vi "Generate SQL Values.vi"(8 "error in (no error)":errorcluster, 11 "Transaction in":refnum<class "Transaction.lvclass">) -> (0 "error out":errorcluster, 2 "SQL Values":string, 3 "Transaction out":refnum<class "Transaction.lvclass">)   [LabVIEW 2018, in "Transaction.lvclass"]
uses:
  Transaction/Transaction.lvclass
  Transaction/Transaction.lvclass/Transaction.ctl
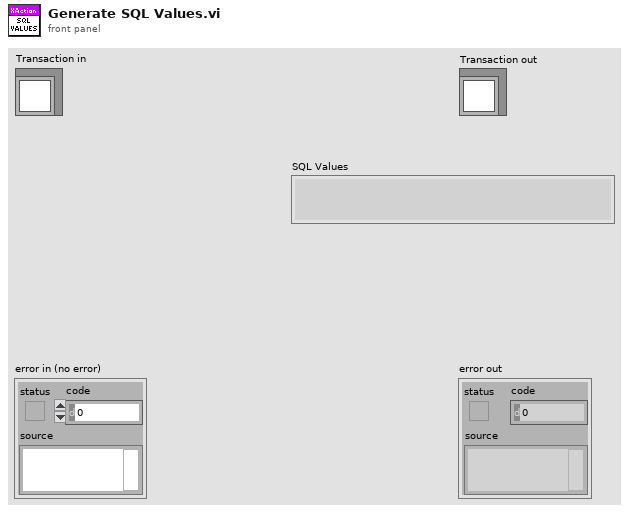
[diagram p1: front panel]
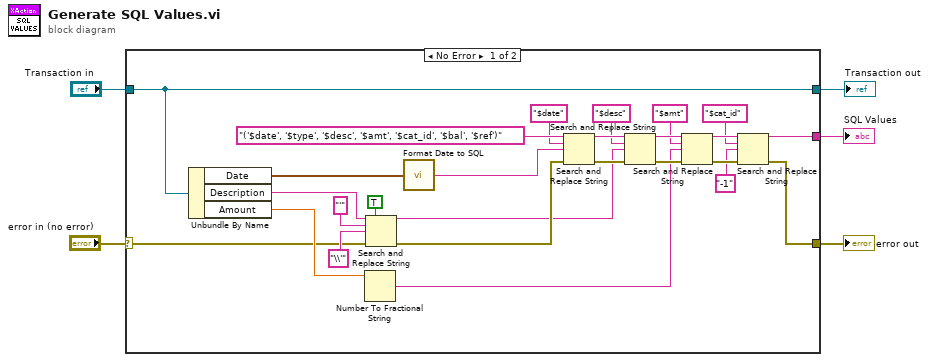
[diagram p0: block diagram]
diagram:
  n1 = case shown="No Error" "error in (no error)" {
    selector: "error in (no error)" -> [w26 w33]
    tunnel: [w13 w33] -> w4
    tunnel: "Transaction in" -> [w25 w32]
    tunnel: [w25 w32] -> w2
    tunnel: [w12 _] -> w1
    frame No Error {
      n2 = Unbundle By Name(w25) -> ("Date"=w24:timestamp, "Description"=w28:string, "Amount"=w27:dbl)
      n3 = Number To Fractional String(number=w27) -> (F-format string=w10:string)  [unwired: 3 in]
      n4 = Search and Replace String(replace all?=TRUE ("replace all? (F)"), input string=w28, search string="'", replace string="\\'", error in=w26) -> (result string=w11:string, error out=w14:errorcluster)  [unwired: 5 out]
      n5 = call "Format Date to SQL.vi"("Date"=w24) -> ("SQL Date"=w21:string)
      n6 = Search and Replace String(input string="('$date', '$type', '$desc', '$amt', '$cat_id', '$bal', '$ref')", search string="$date", replace string=w21, error in=w14) -> (result string=w19:string, error out=w20:errorcluster)  [unwired: 4 in, 2 out]
      n7 = Search and Replace String(input string=w19, search string="$desc", replace string=w11, error in=w20) -> (result string=w18:string, error out=w17:errorcluster)  [unwired: 4 in, 2 out]
      n8 = Search and Replace String(input string=w18, search string="$amt", replace string=w10, error in=w17) -> (result string=w16:string, error out=w15:errorcluster)  [unwired: 4 in, 2 out]
      n9 = Search and Replace String(input string=w16, search string="$cat_id", replace string="-1" ("replace string (\"\")"), error in=w15) -> (result string=w12:string, error out=w13:errorcluster)  [unwired: 4 in, 2 out]
    }
    frame Error {
    }
  }
  "error out" <- w4
  "Transaction out" <- w2
  "SQL Values" <- w1
